vi "Day-02 pt 2 Submarine Navigation.vi"() -> ()   [LabVIEW 2020, in "Advent of Code.lvlib"]
uses:
  Advent of Code.lvlib
panel:
  out "Displacement Product":i32
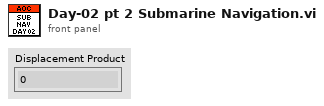
[diagram p1: front panel]
types:
  T1 = typedef "Advent of Code.lvlib/Navigation Command.ctl" = cluster{"Direction":T2, "Value":i32}
  T2 = typedef "Advent of Code.lvlib/Navigation Directions.ctl" = enum16{"forward", "down", "up"}
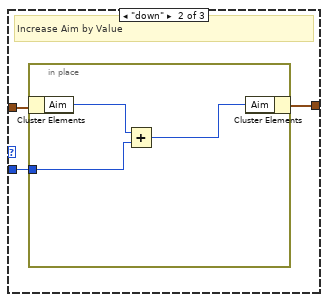
[diagram p2: hidden frame]
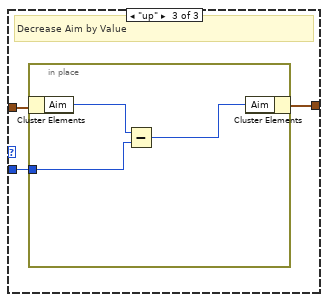
[diagram p3: hidden frame]
diagram:
  # "In addition to horizontal position and depth, you'll also need to track a third value, aim, which also starts at 0. The commands also mean something entirely different than you first thought:\n\ndown X increases your aim by X units.\nup X decreases your aim by X units.\nforward X does two things:\nIt increases your horizontal position by X units.\nIt increases your depth by your aim multiplied by X."
  n1 = call "Parse Navigation Commands.vi"("Input"="forward 5\nforward 1\nforward 3\ndown 8\nup 6\ndown 5\nforward 6\ndown 9\ndown 7\nup 9\ndown 9\nforward 5\nforward 3\ndown 3\nforward 1\nforward 8\ndown 8\nforward 6\nforward 9\nforward 5\ndown 8\nup 1\nforward 4\nforward 8\ndown 4\nforward 2\ndown 1\nup 8\nup 9\ndown 4\nforward 5\nup 9\nforward 1\ndown 9\ndown 7\ndown 4\ndown 6\ndown 3\nforward 5\nup 4\nup 7\nforward 1\ndown 1\nup 3\nforward 8\ndown 8\nup 2\nforward 2\ndown 7\ndown 7\ndown 4\nforward 3\ndown 5\nup 8\ndown 6\nup 2\ndown 7\nforward 8\ndown 7\ndown 7\nup 6\nforward 8\nup 1\ndown 4\nforward 1\ndown 1\ndown 9\ndown 1\ndown 7\nforward 2\nforward 3\nup 8\nup 1\nforward 4\nforward 7\nforward 9\nup 8\ndown 9\ndown 3\ndown 5\ndown 5\nforward 7\nforward 3\nup 7\nforward 6\nup 6\nforward 3\ndown 2\ndown 5\ndown 2\nup 6\ndown 5\ndown 5\nforward 7\nforward 2\nforward 7\ndown 6\nforward 1\nforward 8\nup 6\nforward 2\ndown 5\nforward 3\nup 2\nforward 3\ndown 2\nforward 4\nforward 6\ndown 8\nforward 7\nforward 6\ndown 1\ndown 8\nforward 7\nup 2\nforward 2\ndown 7\nup 6\nforward 7\ndown 9\ndown 7\nforward 4\ndown 9\ndown 4\nforward 6\nup 6\nup 5\ndown 5\nup 7\nforward 6\ndown 1\ndown 5\nforward 1\nup 6\nforward 1\ndown 7\nforward 7\nforward 4\nup 5\ndown 3\nforward 7\nforward 6\nup 9\nforward 8\nforward 1\nup 2\nup 8\nforward 7\nup 7\ndown 1\nforward 9\ndown 5\nforward 5\nforward 2\nforward 2\nforward 6\nup 5\nup 1\nforward 6\nup 3\ndown 7\ndown 6\ndown 1\nforward 1\nforward 8\nforward 8\ndown 8\nup 3\ndown 7\ndown 2\ndown 9\nforward 9\ndown 7\nforward 4\ndown 9\nforward 8\ndown 1\ndown 5\ndown 9\ndown 8\nforward 8\ndown 3\nforward 4\nforward 6\nup 3\nforward 4\ndown 9\ndown 6\nup 6\nup 3\ndown 2\nup 1\nforward 5\ndown 7\ndown 3\nforward 5\nup 1\nforward 2\ndown 3\ndown 3\nforward 6\ndown 5\ndown 7\ndown 1\ndown 2\ndown 7\nforward 4\nforward 7\ndown 7\nforward 6\nforward 2\ndown 1\ndown 8\nforward 5\nforward 5\ndown 7\nforward 6\nforward 7\nup 2\nforward 5\ndown 8\nforward 7\ndown 7\nup 6\nforward 6\ndown 2\ndown 7\nforward 6\nforward 4\ndown 5\ndown 7\nforward 2\nforward 6\nforward 6\ndown 7\ndown 9\nforward 9\nforward 4\nup 9\nup 2\nup 2\nforward 4\ndown 6\nforward 7\nup 5\nforward 1\nforward 6\ndown 8\nforward 2\ndown 8\nforward 9\nforward 5\nforward 1\nup 8\ndown 4\ndown 2\ndown 9\nup 6\nforward 8\ndown 9\nforward 3\ndown 3\ndown 9\ndown 9\ndown 6\nforward 7\ndown 4\nforward 8\ndown 7\ndown 8\nup 4\nup 3\nforward 1\nup 9\nup 1\nup 9\nup 7\ndown 1\nforward 5\nforward 7\nforward 3\nforward 8\nup 4\nforward 7\ndown 5\nforward 9\nup 3\nup 3\ndown 2\nforward 3\nup 3\ndown 3\ndown 4\nup 6\ndown 7\ndown 1\ndown 7\nforward 1\ndown 4\nforward 9\ndown 9\nup 8\nup 5\ndown 7\nup 1\nforward 6\ndown 1\ndown 4\ndown 3\nforward 7\nforward 4\nup 6\ndown 2\ndown 1\nforward 1\nup 5\ndown 2\ndown 9\nup 2\nup 3\nforward 5\nforward 5\ndown 8\ndown 4\nup 4\ndown 1\nforward 8\nup 7\ndown 1\ndown 4\nforward 3\nup 4\ndown 4\ndown 5\ndown 9\ndown 1\ndown 7\nup 2\ndown 6\nup 9\ndown 3\ndown 1\ndown 8\ndown 4\nup 2\nforward 6\nforward 9\ndown 6\nforward 6\nforward 4\nforward 8\nforward 5\nforward 6\nforward 9\ndown 3\nforward 8\nforward 6\nforward 7\nup 9\nforward 3\nup 3\nforward 5\ndown 5\nup 9\nforward 1\nforward 9\ndown 7\nforward 5\nforward 5\nforward 6\nforward 5\nforward 9\nforward 8\nforward 3\ndown 2\nforward 6\nforward 8\ndown 4\nforward 4\nforward 1\nforward 1\ndown 2\nforward 2\nforward 5\nup 4\nforward 3\ndown 3\ndown 5\ndown 6\nforward 4\ndown 8\ndown 4\nforward 5\ndown 7\nup 3\nup 6\nforward 3\nforward 2\nforward 5\ndown 9\ndown 4\ndown 8\ndown 2\nforward 4\nforward 7\ndown 4\nup 5\nforward 8\ndown 8\ndown 1\nforward 5\ndown 6\ndown 9\nup 6\nforward 9\ndown 3\nforward 6\nforward 2\ndown 5\nforward 1\ndown 1\ndown 1\nforward 2\nup 9\ndown 1\nup 8\nforward 9\nup 8\nforward 2\nforward 8\nup 2\nforward 4\ndown 5\nforward 8\nup 2\nup 1\nforward 4\nup 4\nup 3\nup 5\ndown 1\nforward 3\nforward 6\nforward 9\nforward 6\nup 8\nforward 2\nforward 1\ndown 2\ndown 3\ndown 2\nup 4\nforward 5\nup 2\nforward 3\nforward 9\nup 5\nforward 1\ndown 7\nforward 9\ndown 5\nup 7\ndown 6\nforward 7\nforward 9\nup 6\nforward 3\ndown 1\nforward 1\ndown 8\ndown 2\nup 9\ndown 4\ndown 4\ndown 7\nforward 4\nforward 1\nforward 6\ndown 9\ndown 9\ndown 9\nforward 1\nforward 6\nforward 3\nforward 7\nforward 3\nforward 9\nup 8\nforward 5\ndown 1\ndown 6\nup 8\nforward 3\nup 8\ndown 6\nforward 6\nup 2\nup 8\nup 5\nforward 9\ndown 4\nup 1\nup 3\nup 2\ndown 9\ndown 1\nforward 7\ndown 2\nforward 6\nup 4\ndown 7\nforward 1\ndown 3\ndown 5\nforward 1\ndown 3\ndown 1\nforward 8\nup 5\nforward 5\nforward 8\nforward 8\nforward 8\nforward 2\ndown 3\ndown 6\nup 2\nup 2\ndown 1\nup 7\ndown 9\nup 1\nup 4\nforward 1\nforward 4\nup 4\nup 6\nforward 5\nforward 2\nforward 7\nup 8\nup 3\ndown 5\ndown 9\nforward 4\nforward 5\nforward 5\ndown 1\nup 8\nup 2\nforward 3\nup 2\nforward 8\nup 2\ndown 6\nup 7\nforward 6\ndown 3\nforward 3\ndown 6\nforward 6\nforward 4\nforward 8\ndown 8\nup 7\ndown 7\ndown 2\nup 5\nup 2\ndown 4\nforward 5\ndown 3\nup 4\ndown 2\nup 2\ndown 7\nforward 4\nforward 3\nforward 6\ndown 2\ndown 8\nforward 3\nforward 4\nforward 4\ndown 4\ndown 3\nup 6\ndown 2\nforward 7\nforward 4\ndown 7\nforward 1\nup 6\nforward 3\nup 3\nup 7\nforward 6\ndown 9\ndown 8\ndown 3\nforward 8\nforward 1\nup 3\ndown 5\ndown 3\nforward 1\nup 9\ndown 6\nforward 3\ndown 9\nup 7\nforward 5\nforward 4\nforward 7\nup 3\nforward 3\ndown 5\nforward 7\nforward 9\ndown 6\nforward 7\nforward 5\nup 6\nforward 3\nforward 3\ndown 7\nforward 4\nup 2\nforward 8\ndown 7\nup 7\ndown 7\nforward 6\nup 3\nforward 2\nup 7\ndown 3\ndown 4\ndown 1\nforward 3\nforward 5\nup 7\nforward 3\ndown 1\ndown 2\nup 4\nforward 2\nup 5\ndown 4\nforward 1\ndown 6\nup 1\nforward 5\nforward 1\ndown 8\nforward 7\ndown 7\nforward 4\nforward 7\nforward 3\nforward 2\nforward 1\nforward 7\ndown 1\nforward 9\nforward 9\nforward 8\nforward 9\nforward 8\nforward 5\nforward 1\nup 5\nforward 3\nforward 6\nforward 1\nup 4\ndown 1\ndown 9\ndown 6\nforward 4\nup 9\ndown 3\nforward 2\ndown 3\nup 2\nforward 4\nforward 4\ndown 7\nforward 9\nforward 3\ndown 4\nup 4\ndown 4\nforward 7\nforward 3\nforward 6\nforward 9\ndown 4\ndown 5\ndown 2\nforward 4\nup 6\nforward 8\nforward 3\ndown 2\ndown 5\nforward 4\ndown 8\nup 5\ndown 3\nforward 6\ndown 8\nup 9\nforward 3\nforward 8\nforward 6\nforward 7\ndown 3\nup 6\ndown 7\ndown 4\nforward 2\nforward 5\ndown 1\ndown 5\ndown 5\nforward 6\nforward 6\ndown 1\nforward 2\nup 1\ndown 2\ndown 3\nforward 3\nforward 9\ndown 9\ndown 1\nup 8\ndown 5\ndown 2\nup 7\nforward 8\nup 7\nforward 3\nforward 6\ndown 2\ndown 3\nforward 1\ndown 6\ndown 1\nforward 4\nup 2\ndown 3\nup 7\ndown 3\ndown 2\nup 8\nup 7\ndown 3\nforward 4\ndown 8\nup 2\ndown 6\nforward 9\ndown 1\nup 3\nup 1\ndown 4\nup 6\ndown 2\nforward 1\ndown 6\nforward 4\nforward 3\ndown 7\ndown 2\ndown 6\ndown 2\ndown 7\nforward 2\ndown 1\nup 8\nup 6\nup 1\nforward 5\ndown 9\ndown 5\nup 7\ndown 4\nforward 4\nforward 5\nup 5\nforward 6\nforward 1\nforward 5\nforward 1\nforward 6\ndown 6\nforward 3\nup 4\nforward 6\ndown 6\nforward 1\nforward 5\nforward 8\ndown 3\nforward 6\nforward 1\nup 1\nup 7\nforward 7\nforward 8\nup 6\nforward 9\nup 5\nforward 1\nforward 5\ndown 3\nup 3\nup 9\nforward 9\nforward 5\nforward 3\nforward 2\nforward 4\ndown 6\nup 5\ndown 2\nforward 5\ndown 2\ndown 5\ndown 6\nforward 7\ndown 2\nforward 7\nforward 2\nforward 8\nup 1\nforward 9\ndown 2\nup 1\ndown 9\nforward 8\nforward 3\nup 9\ndown 1\ndown 1\ndown 8\nup 4\nup 9\nforward 9\nforward 3\ndown 9\nforward 3\nforward 4\ndown 8\nforward 8\nforward 7\ndown 9\nup 2\ndown 9\ndown 8\ndown 9\nforward 4\nup 6\ndown 4\nforward 8\nforward 5\nup 2\nforward 5\ndown 3\nforward 6\ndown 5\nforward 8\nup 3\ndown 5\ndown 4\nforward 5\nup 3\nup 8\nforward 1\nup 8\nforward 4\ndown 4\nforward 7\nforward 5\nforward 7\nforward 9\nup 1\ndown 6\nforward 8\nup 1\ndown 5\nup 6\ndown 9\ndown 5\nforward 3\nup 1\nforward 4\nup 4\ndown 4\nforward 5\nforward 8\ndown 2\nup 7\ndown 6\nforward 7\nup 7\nforward 5\ndown 2\nforward 9\nforward 1\ndown 9\ndown 8\nforward 7\nforward 7\nforward 1\nup 3\nup 1\nforward 2\ndown 2\nup 9\ndown 2\nforward 7\ndown 1\ndown 5\ndown 4\nup 7\nforward 1\ndown 3\nforward 9\ndown 6\nforward 4\ndown 4\ndown 9\ndown 3\nup 3\ndown 3\nup 8\ndown 2\nforward 1\nforward 5\nforward 5\ndown 2\nforward 7\ndown 7\ndown 6\nforward 6\nup 5\ndown 4\ndown 8\ndown 7\nforward 7\nup 3\ndown 3\ndown 3\nforward 8\nforward 5\ndown 1\nup 6\ndown 3\nup 2\ndown 6\nup 7\ndown 4\nup 2\nforward 4\nforward 9\nforward 9\nup 1\nforward 7\nup 7\nforward 7\nforward 6\nforward 3\nforward 1\ndown 5\ndown 3\nforward 4\nup 9\ndown 5\nup 2\ndown 6\ndown 5\nforward 6\nforward 4\nup 7\nup 6\ndown 9\nforward 4\nup 1\nup 6\nup 3\nforward 9\nforward 3\nforward 9\ndown 7\nforward 6\ndown 6\nforward 8") -> ("Commands"=w6:T1[])  [unwired: 9 in, 1 out]
  n2 = for {
    tunnel: w6 -> [w12] mode=indexing
    shift-right: [w8] -> w4
    shift-left: cluster{"Depth":i32, "Position":i32, "Aim":i32} {"Depth"=0, "Position"=0, "Aim"=0} -> [w9]
    n3 = Unbundle By Name(w12) -> ("Direction"=w11:T2, "Value"=w10:i32)
    n4 = case shown="\"forward\"" w11 {
      tunnel: w10 -> [w14 w24 w30]
      tunnel: w9 -> [w15 w25 w31]
      tunnel: [w13 w23 w29] -> w8
      frame "forward" {
        # "Increase Position by Value\nIncrease Depth by (Aim * Value)"
        n5 = in-place {
          in-place-border: w14 -> [w19]
          n6 = in-place-cluster #1(w15) -> ("Aim"=w20:i32, "Position"=w22:i32, "Depth"=w17:i32)
          n7 = Add(x=w22, y=w19) -> (x+y=w21:i32)
          n8 = Multiply(x=w20, y=w19) -> (x*y=w18:i32)
          n9 = Add(x=w17, y=w18) -> (x+y=w16:i32)
          n10 = in-place-cluster #1("Aim"=w20, "Position"=w21, "Depth"=w16) -> (w13:cluster{"Depth":i32, "Position":i32, "Aim":i32})
        }
      }
      frame "down" {
        # "Increase Aim by Value"
        n11 = in-place {
          in-place-border: w24 -> [w28]
          n12 = in-place-cluster #2(w25) -> ("Aim"=w27:i32)
          n13 = Add(x=w27, y=w28) -> (x+y=w26:i32)
          n14 = in-place-cluster #2("Aim"=w26) -> (w23:cluster{"Depth":i32, "Position":i32, "Aim":i32})
        }
      }
      frame "up" {
        # "Decrease Aim by Value"
        n15 = in-place {
          in-place-border: w30 -> [w34]
          n16 = in-place-cluster #3(w31) -> ("Aim"=w33:i32)
          n17 = Subtract(x=w33, y=w34) -> (x-y=w32:i32)
          n18 = in-place-cluster #3("Aim"=w32) -> (w29:cluster{"Depth":i32, "Position":i32, "Aim":i32})
        }
      }
    }
  }
  n19 = Unbundle By Name(w4) -> ("Depth"=w3:i32, "Position"=w2:i32)
  n20 = Multiply(x=w3, y=w2) -> (x*y=→"Displacement Product":i32)
